vi "testSendTel.vi"(8 "error in (no error)":errorcluster) -> (0 "error out":errorcluster)   [LabVIEW 2018]
doc: "Test the sendTel.vi."
uses:
  src/TcpServer/TcpServer.lvclass
  src/TcpServerBase/typedef/msgTypeDef.ctl
  src/TcpServerTel/typedef/queueOptionsTypeDef.ctl
  src/TcpServerTel/typedef/enqueueOptionsTypeDef.ctl
  src/TcpServer/TcpServer.lvclass/TcpServer.ctl
  src/TcpServerBase/TcpServerBase.lvclass/TcpServerBase.ctl
  src/TcpServerTel/TcpServerTel.lvclass
  home/pcortes/github/ts_labview_tcp_json/src/TcpServerBase/TcpServerBase.lvclass
  <vilib>/addons/_JKI Toolkits/Caraya/classes/Assert/Assert Equal Value_Variant.vi
  <vilib>/addons/_JKI Toolkits/Caraya/classes/Test/Test.lvclass
  <vilib>/addons/_JKI Toolkits/Caraya/classes/Assert/Assert.lvclass
  src/TcpServerBase/TcpServerBase.lvclass
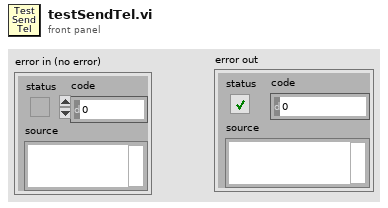
[diagram p1: front panel]
types:
  T1 = typedef "TcpServerTel.lvclass/queueOptionsTypeDef.ctl" = cluster{"EnqueueOptions":T2, "Timeout (ms)":i32}
  T2 = typedef "TcpServerTel.lvclass/enqueueOptionsTypeDef.ctl" = enum16{"lossy enqueue", "normal enqueue"}
  T3 = typedef "TcpServerBase.lvclass/msgTypeDef.ctl" = cluster{"msgName":string, "msgDetails":string}
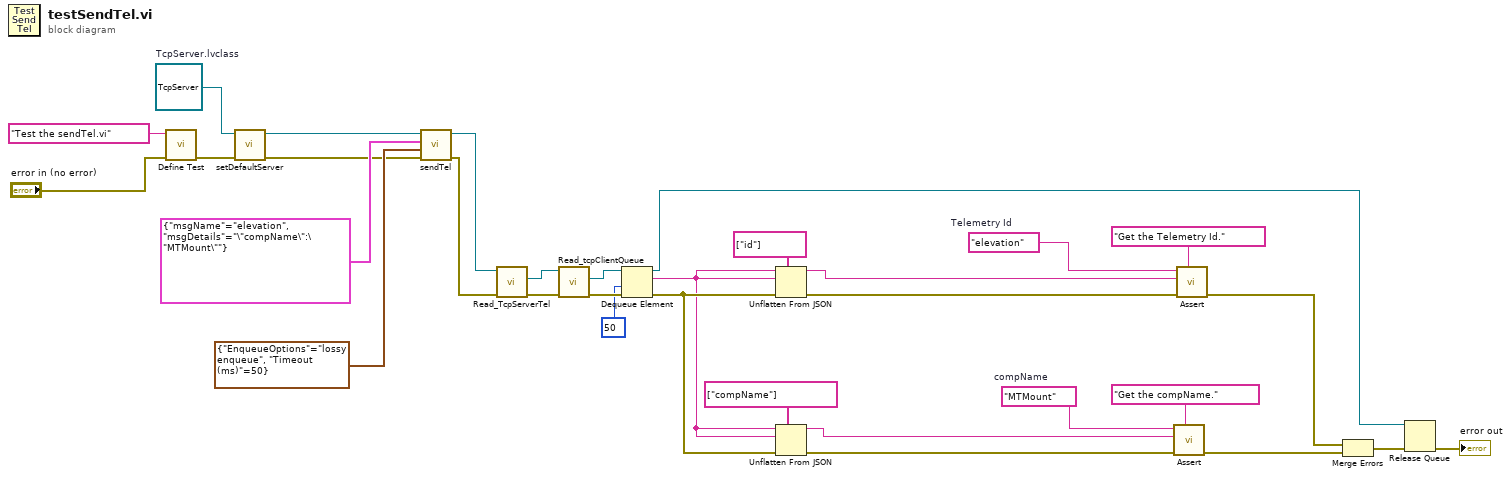
[diagram p0: block diagram]
diagram:
  w8 = "MTMount"  # compName
  w9 = "elevation"  # Telemetry Id
  w29 = refnum<class "TcpServer.lvclass"> refnum  # TcpServer.lvclass
  n1 = call <vilib>:"Define Test.vi"("error in (no error)"="error in (no error)", "Label (VI Title)"="Test the sendTel.vi") -> ("error out"=w31:errorcluster)  [unwired: 9 in]
  n2 = call "setDefaultServer.vi"("error in (no error)"=w31, "TcpServer.lvclass"=w29) -> ("error out"=w25:errorcluster, "tcpServer out"=w28:refnum<class "TcpServer.lvclass">)  [unwired: 8 in]
  n3 = call "sendTel.vi"("error in (no error)"=w25, "queueOptions"=T1 {"EnqueueOptions"=enum."lossy enqueue", "Timeout (ms)"=50}, "Telemetry"=T3 {"msgName"="elevation", "msgDetails"="\"compName\":\"MTMount\""} ("telData"), "tcpServer in"=w28) -> ("error out"=w18:errorcluster, "tcpServer out"=w19:refnum<class "TcpServer.lvclass">)  [unwired: 6 in]
  n4 = call "Read_TcpServerTel.vi"("error in (no error)"=w18, "TcpServer in"=w19) -> ("error out"=w24:errorcluster, "TcpServerTel.lvclass"=w23:refnum<class "TcpServerTel.lvclass">)  [unwired: 7 in, 1 out]
  n5 = call "Read_tcpClientQueue.vi"("error in (no error)"=w24, "TcpServerBase in"=w23) -> ("error out"=w22:errorcluster, "tcpClientQueue"=w21:refnum<queue>)  [unwired: 7 in, 1 out]
  n6 = Dequeue Element(queue=w21, timeout in ms (-1)=50, error in (no error)=w22) -> (queue out=w1:refnum<queue>, element=w16:string, error out=w17:errorcluster)  [unwired: 1 out]
  n7 = Unflatten From JSON(path=string[] ["id"], JSON string=w16, type and defaults=w16, error in (no error)=w17) -> (value=w7:string, error out=w6:errorcluster)  [unwired: 3 in]
  n8 = Unflatten From JSON(path=string[] ["compName"], JSON string=w16, type and defaults=w16, error in (no error)=w17) -> (value=w4:string, error out=w5:errorcluster)  [unwired: 3 in]
  n9 = call-poly <vilib>:"Assert.vi"("Label"="Get the compName.", "error in (no error)"=w5, "Y"=w4, "X"=w8) -> ("error out"=w11:errorcluster)  [unwired: 7 in]
  n10 = call-poly <vilib>:"Assert.vi"("Label"="Get the Telemetry Id.", "error in (no error)"=w6, "Y"=w7, "X"=w9) -> ("error out"=w10:errorcluster)  [unwired: 7 in]
  n11 = Merge Errors(w10, w11) -> (w3:errorcluster)
  n12 = Release Queue(queue=w1, error in (no error)=w3) -> (error out=→"error out":errorcluster)  [unwired: 1 in, 2 out]
